vi "Set global var.vi"(8 "error in (no error)":errorcluster, 9 "New key data":string, 10 "Key Name":string="test_pc_name", 11 "Section Name":string="general") -> (0 "error out":errorcluster, 3 "KeyFound?":bool)   [LabVIEW 2013]
doc: "Gets key data from global.ini file in exe directory"
uses:
  Test Globals/Global 1.vi
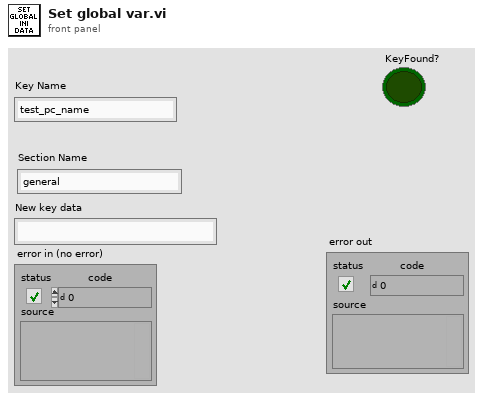
[diagram p1: front panel]
types:
  T1 = enum16{"Read config file key", "Write config file key", "Read config file key and compare"}
  T2 = cluster{"Test folder":string, "Top level":string, "Main":string, "Test report":string, "Work order qty":string, "Work order meid":string, "Work order imei":string, "Master meid imei list":string, "Master test data":string, "ZPL label info":string, "Pictures":string, "Setup info":string, "Work order":string, "Tests folder":string, "Tests steps folder":string, "Config folder":string, "Verizon Upload file":string, "Job data file":string, "Station globals":string, "Post test info":string}
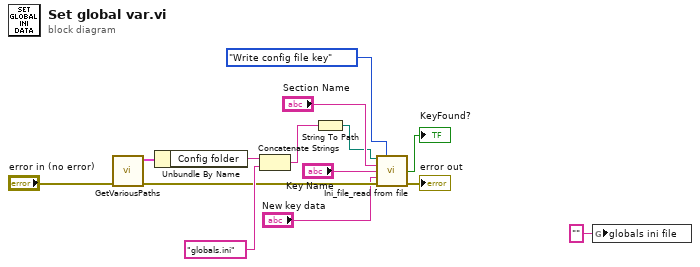
[diagram p0: block diagram]
diagram:
  n1 = call "GetVariousPaths.vi"("error in (no error)"="error in (no error)") -> ("error out"=w6:errorcluster, "Built Paths"=w9:T2)  [unwired: 9 in]
  n2 = Unbundle By Name(w9) -> ("Config folder"=w8:string)
  n3 = Concatenate Strings(w8, "globals.ini" ("string")) -> (w11:string)
  n4 = String To Path(string=w11) -> (path=w3:path)
  n5 = call "Ini_file_read from file.vi"("config file path"=w3, "Operation"=T1."Write config file key", "Section Name"="Section Name", "Key Name"="Key Name", "New key data"="New key data", "error in (no error)"=w6) -> ("KeyFound?"=→"KeyFound?":bool, "error out"=→"error out":errorcluster)  [unwired: 6 in, 2 out]
  n6 = global write "Global 1.vi" "globals ini file"("" ("globals ini file")) -> ()
